vi "WfgConfigureSweepCh1.vi"(0 "object in":refnum<class "AD2_WFG_SDK.lvclass">, 2 "Sweep Settings":T1={"Ch1"={"Ch.Carrier.Enable"=FALSE, "Ch.Center Frequency(Hz)"=0.0, "Ch.Carrier.Amplitude (V)"=0.0, "Function"=5, "Ch Sweep Width (% of Center Freq)"=0.0, "Sweep Repetition Rate (Hz)"=0.0, "Sweep Type"=enum."Symmetric", "Enable Sweep"=FALSE}, "Ch2"={"Ch.Carrier.Enable"=FALSE, "Ch.Center Frequency(Hz)"=0.0, "Ch.Carrier.Amplitude (V)"=0.0, "Function"=5, "Ch Sweep Width (% of Center Freq)"=0.0, "Sweep Repetition Rate (Hz)"=0.0, "Sweep Type"=enum."Symmetric", "Enable Sweep"=FALSE}} {"Ch2"."Function" items=["DC"=0, "Sine"=1, "Square"=2, "Triangle"=3, "RampUp"=4, "RampDown"=5, "Noise"=6, "Pulse"=7, "Custom"=30]; "Ch1"."Function" items=["DC"=0, "Sine"=1, "Square"=2, "Triangle"=3, "RampUp"=4, "RampDown"=5, "Noise"=6, "Pulse"=7, "Custom"=30]}, 5 "error in (no error)":errorcluster) -> (14 "object out":refnum<class "AD2_WFG_SDK.lvclass">, 15 "Ch1 Top Frequency(Hz)":dbl, 16 "Ch1 Bottom Frequency(Hz)":dbl, 17 "Ch2 Top Frequency(Hz)":dbl, 18 "Ch2 Bottom Frequency(Hz)":dbl, 19 "error out":errorcluster)   [LabVIEW 2019, in "AD2_WFG_SDK.lvclass"]
uses:
  AD2_WFG_SDK.lvclass
  BasicSweepSettings.ctl
  WFGCh.ctl
  AD2TriggerSources.ctl
  AD2_WFG_SDK.lvclass/AD2_WFG_SDK.ctl
  AD2_SDK_class/AD2_SDK.lvclass
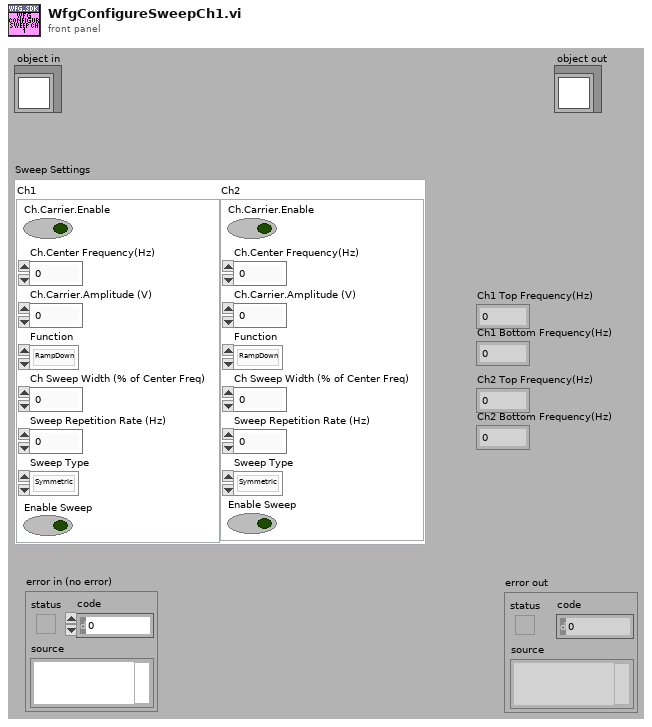
[diagram p1: front panel]
types:
  T1 = typedef "AD2_WFG_SDK.lvclass/BasicSweepSettings.ctl" = cluster{"Ch1":cluster{"Ch.Carrier.Enable":bool, "Ch.Center Frequency(Hz)":dbl, "Ch.Carrier.Amplitude (V)":dbl, "Function":u16, "Ch Sweep Width (% of Center Freq)":dbl, "Sweep Repetition Rate (Hz)":dbl, "Sweep Type":enum16{"Symmetric", "RampUp", "RampDown"}, "Enable Sweep":bool}, "Ch2":cluster{"Ch.Carrier.Enable":bool, "Ch.Center Frequency(Hz)":dbl, "Ch.Carrier.Amplitude (V)":dbl, "Function":u16, "Ch Sweep Width (% of Center Freq)":dbl, "Sweep Repetition Rate (Hz)":dbl, "Sweep Type":enum16{"Symmetric", "RampUp", "RampDown"}, "Enable Sweep":bool}}
  T2 = typedef "AD2_WFG_SDK.lvclass/WFGCh.ctl" = cluster{"idxChannel":i32, "Settings out of range":bool, "Carrier":cluster{"Frequency (Hz)":dbl, "Amplitude (V)":dbl, "Offset(V)":dbl, "Symmetry(%) ":dbl, "Phase(Deg)":dbl, "Function":u16, "Enable":bool}, "Trigger":cluster{"secRun(0=Cont)":dbl, "secWait":dbl, "cRepeat(0=inf)":i32, "Repeat Trigger":bool, "TrigrSrc":T3}, "FM Mod":cluster{"Frequency (Hz)":dbl, "Amplitude (%)":dbl, "Offset(V)":dbl, "Symmetry(%) ":dbl, "Phase(Deg)":dbl, "Function 2":u16, "Enable":bool}}
  T3 = typedef "AD2_SDK.lvclass/AD2TriggerSources.ctl" = enum8{"trigrsrcNone", "trigsrcPC", "trigsrcDetectorAnalogIn", "trigsrcDetectorDigitalIn", "trigsrcAnalogIn", "trigsrcDigitalIn", "trigsrcDigitalOut", "trigsrcAnalogOut1", "trigsrcAnalogOut2", "trigsrcAnalogOut3", "trigsrcAnalogOut4", "trigsrcExternal1", "trigsrcExternal2", "trigsrcExternal3", "trigsrcExternal4", ""}
  T4 = cluster{"Ch.Carrier.Enable":bool, "Ch.Center Frequency(Hz)":dbl, "Ch.Carrier.Amplitude (V)":dbl, "Function":u16, "Ch Sweep Width (% of Center Freq)":dbl, "Sweep Repetition Rate (Hz)":dbl, "Sweep Type":enum16{"Symmetric", "RampUp", "RampDown"}, "Enable Sweep":bool}
  T5 = typedef "AD2_WFG_SDK.lvclass/WFG.ctl" = cluster{"Running":bool, "Ch1":T2, "Ch2":T2, "SyncronizeState":enum16{"Independent", "Ch1Master", "Ch2Master"}}
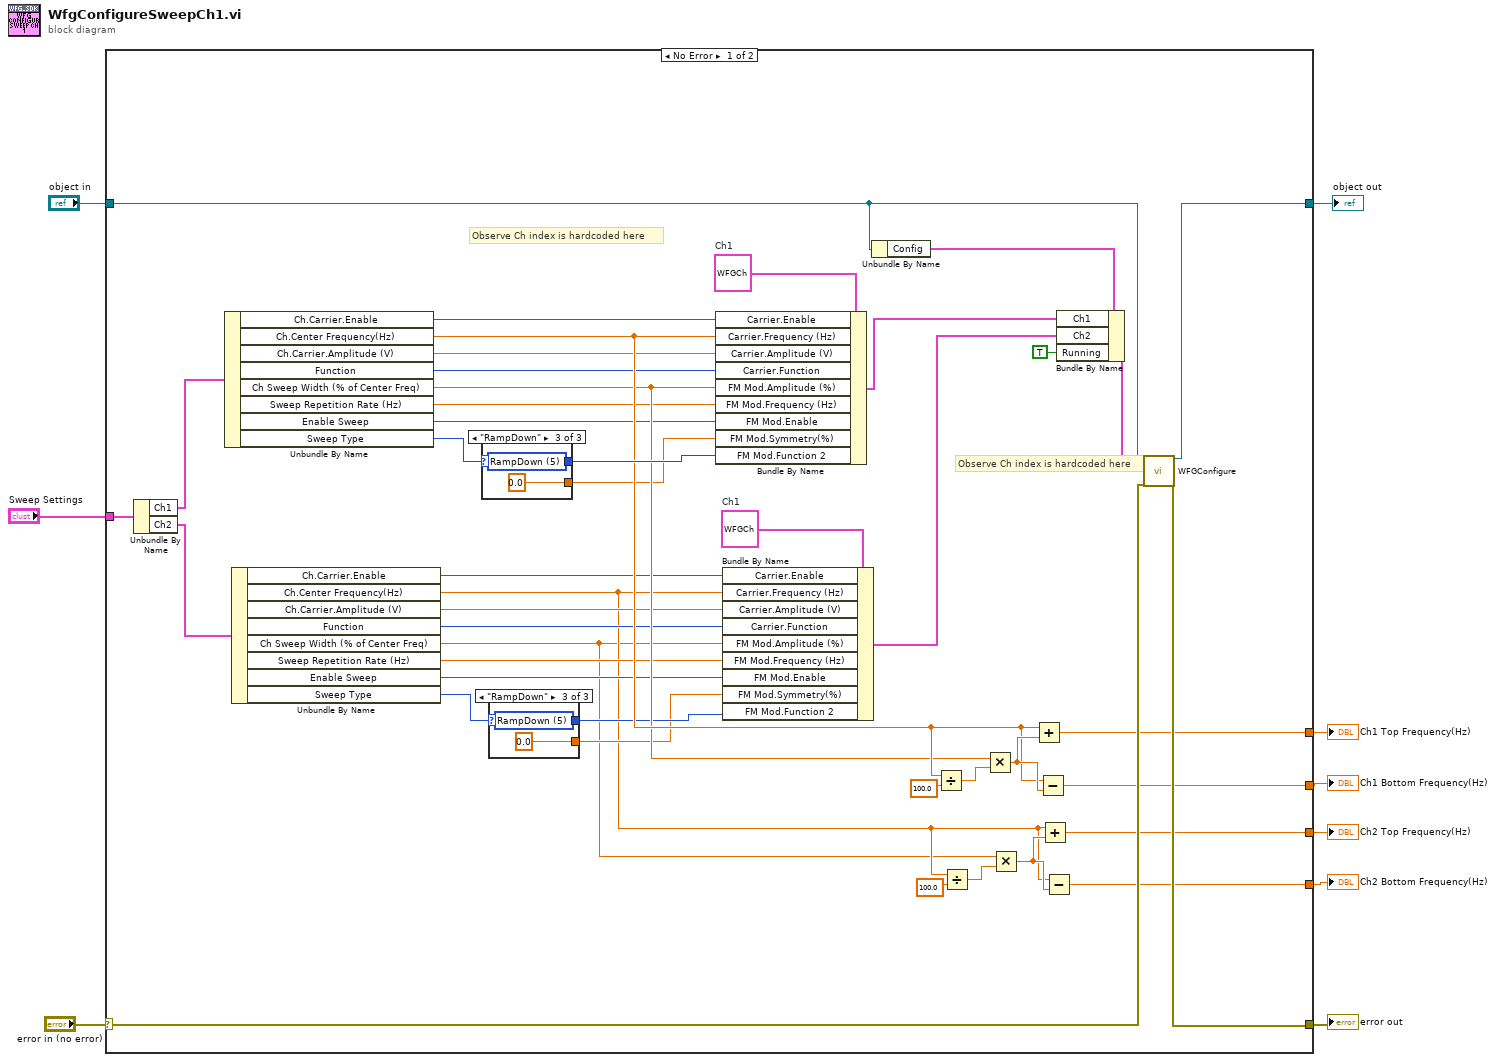
[diagram p0: block diagram]
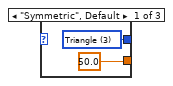
[diagram p2: hidden frame]
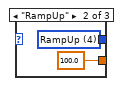
[diagram p3: hidden frame]
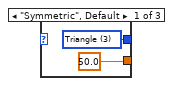
[diagram p4: hidden frame]
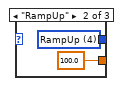
[diagram p5: hidden frame]
diagram:
  n1 = case shown="No Error" "error in (no error)" {
    selector: "error in (no error)" -> [w53 w67]
    tunnel: [w52 w67] -> w8
    tunnel: [w51 w66] -> w6
    tunnel: "object in" -> [w32 w66]
    tunnel: [w46 _] -> w5
    tunnel: [w45 _] -> w4
    tunnel: "Sweep Settings" -> [w30 _]
    tunnel: [w16 _] -> w1
    tunnel: [w17 _] -> w2
    frame No Error {
      w20 = T2 {"idxChannel"=1, "Settings out of range"=FALSE, "Carrier"={"Frequency (Hz)"=0.0, "Amplitude (V)"=1.0, "Offset(V)"=0.0, "Symmetry(%) "=50.0, "Phase(Deg)"=0.0, "Function"=0, "Enable"=FALSE}, "Trigger"={"secRun(0=Cont)"=0.0, "secWait"=0.0, "cRepeat(0=inf)"=0, "Repeat Trigger"=FALSE, "TrigrSrc"=enum."trigrsrcNone"}, "FM Mod"={"Frequency (Hz)"=1000.0, "Amplitude (%)"=1.0, "Offset(V)"=0.0, "Symmetry(%) "=50.0, "Phase(Deg)"=0.0, "Function 2"=1, "Enable"=FALSE}}  # Ch1
      w33 = T2 {"idxChannel"=0, "Settings out of range"=FALSE, "Carrier"={"Frequency (Hz)"=0.0, "Amplitude (V)"=1.0, "Offset(V)"=0.0, "Symmetry(%) "=50.0, "Phase(Deg)"=0.0, "Function"=0, "Enable"=FALSE}, "Trigger"={"secRun(0=Cont)"=0.0, "secWait"=0.0, "cRepeat(0=inf)"=0, "Repeat Trigger"=FALSE, "TrigrSrc"=enum."trigrsrcNone"}, "FM Mod"={"Frequency (Hz)"=1000.0, "Amplitude (%)"=1.0, "Offset(V)"=0.0, "Symmetry(%) "=50.0, "Phase(Deg)"=0.0, "Function 2"=1, "Enable"=FALSE}}  # Ch1
      # "Observe Ch index is hardcoded here"
      # "Observe Ch index is hardcoded here"
      n2 = Unbundle By Name(w30) -> ("Ch1"=w29:T4, "Ch2"=w19:T4)
      n3 = Unbundle By Name(w29) -> ("Ch.Carrier.Enable"=w34:bool, "Ch.Center Frequency(Hz)"=w42:dbl, "Ch.Carrier.Amplitude (V)"=w41:dbl, "Function"=w40:u16, "Ch Sweep Width (% of Center Freq)"=w39:dbl, "Sweep Repetition Rate (Hz)"=w38:dbl, "Enable Sweep"=w35:bool, "Sweep Type"=w36:enum16{"Symmetric", "RampUp", "RampDown"})
      n4 = Unbundle By Name(w19) -> ("Ch.Carrier.Enable"=w21:bool, "Ch.Center Frequency(Hz)"=w12:dbl, "Ch.Carrier.Amplitude (V)"=w27:dbl, "Function"=w26:u16, "Ch Sweep Width (% of Center Freq)"=w11:dbl, "Sweep Repetition Rate (Hz)"=w25:dbl, "Enable Sweep"=w22:bool, "Sweep Type"=w23:enum16{"Symmetric", "RampUp", "RampDown"})
      n5 = case shown="\"RampDown\"" w36 {
        tunnel: [50.0 ("Ch1.FM Mod.Symmetry(%)") 100.0 ("Ch1.FM Mod.Symmetry(%)") 0.0 ("Ch1.FM Mod.Symmetry(%)")] -> w37
        tunnel: [w60 w62 w64] -> w50
        frame "Symmetric", Default {
          w60 = u16 3 items=["DC"=0, "Sine"=1, "Square"=2, "Triangle"=3, "RampUp"=4, "RampDown"=5, "Noise"=6, "Pulse"=7, "Custom"=30] ("Function 2")
        }
        frame "RampUp" {
          w62 = u16 4 items=["DC"=0, "Sine"=1, "Square"=2, "Triangle"=3, "RampUp"=4, "RampDown"=5, "Noise"=6, "Pulse"=7, "Custom"=30] ("Function 2")
        }
        frame "RampDown" {
          w64 = u16 5 items=["DC"=0, "Sine"=1, "Square"=2, "Triangle"=3, "RampUp"=4, "RampDown"=5, "Noise"=6, "Pulse"=7, "Custom"=30] ("Function 2")
        }
      }
      n6 = case shown="\"RampDown\"" w23 {
        tunnel: [50.0 ("Ch1.FM Mod.Symmetry(%)") 100.0 ("Ch1.FM Mod.Symmetry(%)") 0.0 ("Ch1.FM Mod.Symmetry(%)")] -> w24
        tunnel: [w54 w56 w58] -> w28
        frame "Symmetric", Default {
          w54 = u16 3 items=["DC"=0, "Sine"=1, "Square"=2, "Triangle"=3, "RampUp"=4, "RampDown"=5, "Noise"=6, "Pulse"=7, "Custom"=30] ("Function 2")
        }
        frame "RampUp" {
          w56 = u16 4 items=["DC"=0, "Sine"=1, "Square"=2, "Triangle"=3, "RampUp"=4, "RampDown"=5, "Noise"=6, "Pulse"=7, "Custom"=30] ("Function 2")
        }
        frame "RampDown" {
          w58 = u16 5 items=["DC"=0, "Sine"=1, "Square"=2, "Triangle"=3, "RampUp"=4, "RampDown"=5, "Noise"=6, "Pulse"=7, "Custom"=30] ("Function 2")
        }
      }
      n7 = Bundle By Name(cluster=w33, "Carrier.Enable"=w34, "Carrier.Frequency (Hz)"=w42, "Carrier.Amplitude (V)"=w41, "Carrier.Function"=w40, "FM Mod.Amplitude (%)"=w39, "FM Mod.Frequency (Hz)"=w38, "FM Mod.Enable"=w35, "FM Mod.Symmetry(%)"=w37, "FM Mod.Function 2"=w50) -> (w44:T2)
      n8 = Bundle By Name(cluster=w20, "Carrier.Enable"=w21, "Carrier.Frequency (Hz)"=w12, "Carrier.Amplitude (V)"=w27, "Carrier.Function"=w26, "FM Mod.Amplitude (%)"=w11, "FM Mod.Frequency (Hz)"=w25, "FM Mod.Enable"=w22, "FM Mod.Symmetry(%)"=w24, "FM Mod.Function 2"=w28) -> (w18:T2)
      n9 = Unbundle By Name(w32) -> ("Config"=w31:T5)
      n10 = Divide(x=w42, y=100.0) -> (x/y=w48:dbl)
      n11 = Divide(x=w12, y=100.0) -> (x/y=w14:dbl)
      n12 = Multiply(x=w39, y=w48) -> (x*y=w47:dbl)
      n13 = Multiply(x=w11, y=w14) -> (x*y=w15:dbl)
      n14 = Add(x=w42, y=w47) -> (x+y=w46:dbl)
      n15 = Subtract(x=w42, y=w47) -> (x-y=w45:dbl)
      n16 = Add(x=w12, y=w15) -> (x+y=w16:dbl)
      n17 = Subtract(x=w12, y=w15) -> (x-y=w17:dbl)
      n18 = Bundle By Name(cluster=w31, "Ch1"=w44, "Ch2"=w18, "Running"=TRUE) -> (w43:T5)
      n19 = call-dynamic "WFGConfigure.vi"("object in"=w32, "WFGConfig"=w43, "error in (no error)"=w53) -> ("object out"=w51:refnum<class "AD2_WFG_SDK.lvclass">, "error out"=w52:errorcluster)  [unwired: 14 in, 1 out]
    }
    frame Error {
    }
  }
  "error out" <- w8
  "object out" <- w6
  "Ch1 Top Frequency(Hz)" <- w5
  "Ch1 Bottom Frequency(Hz)" <- w4
  "Ch2 Top Frequency(Hz)" <- w1
  "Ch2 Bottom Frequency(Hz)" <- w2
